vi "GetExampleModulePath.vi"() -> (3 "module path":path)   [LabVIEW 2019]
doc: "Helper VI to compute the path of the module used by the Python examples."
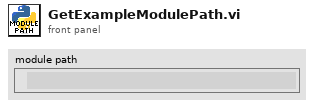
[diagram p1: front panel]
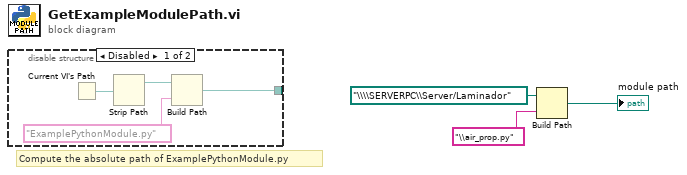
[diagram p0: block diagram]
diagram:
  # "Compute the absolute path of ExamplePythonModule.py"
  n1 = disable-structure shown="Disabled" {
    disable-tunnel: [w4 _] -> _
    frame Disabled {
      n2 = Current VI's Path() -> (path=w7:path)
      n3 = Strip Path(path=w7) -> (stripped path=w6:path)  [unwired: 1 out]
      n4 = Build Path(base path=w6, name or relative path="ExamplePythonModule.py") -> (appended path=w4:path)
    }
    frame Enabled {
    }
  }
  n5 = Build Path(base path=path "\\\\SERVERPC\\Server/Laminador", name or relative path="\\air_prop.py") -> (appended path=→"module path":path)
